vi "fitting.vi"() -> ()   [LabVIEW 2021]
uses:
  <vilib>/Utility/file.llb/Read Delimited Spreadsheet (DBL).vi
  <vilib>/Analysis/NI_AALPro.lvlib
panel:
  out "XY Graph 2":T1(graph)
  in  "path 2":path
  out "XY Graph":T1(graph)
  in  "path":path
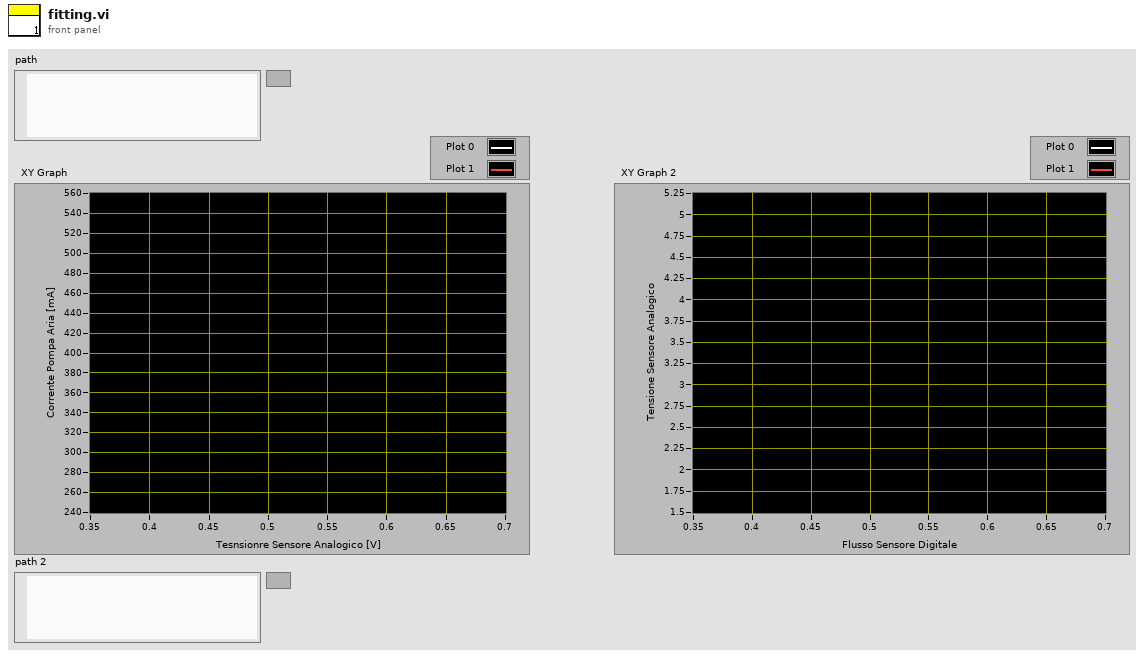
[diagram p1: front panel]
types:
  T1 = cluster{"all rows":dbl[], "Best Polynomial Fit":dbl[]}[]
  T2 = cluster{"all rows":dbl[], "Best Linear Fit":dbl[]}
  T3 = cluster{"all rows":dbl[], "Best Polynomial Fit":dbl[]}
  T4 = cluster{"all rows":dbl[], "Best Linear Fit":dbl[]}[]
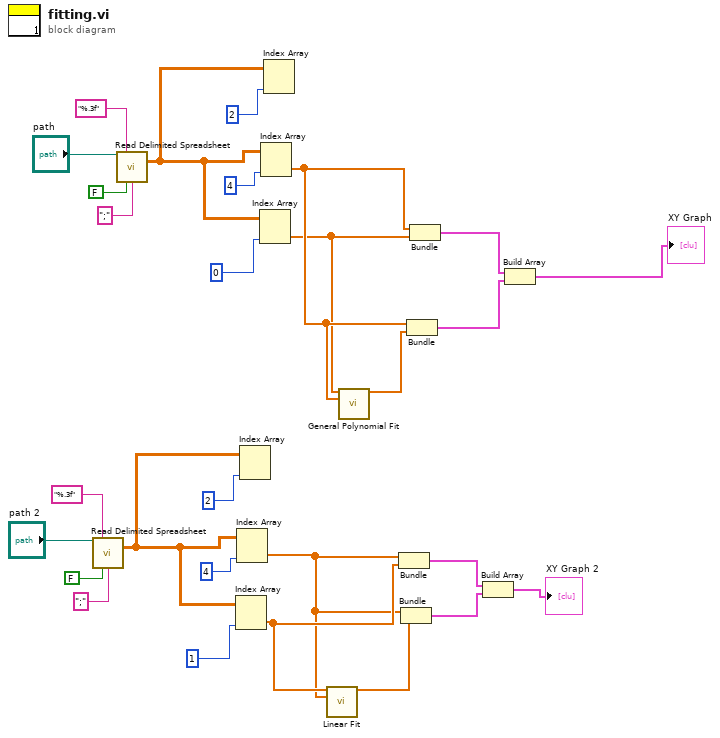
[diagram p0: block diagram]
diagram:
  n1 = call-poly <vilib>:"Read Delimited Spreadsheet.vi"("file path (dialog if empty)"="path 2", "format (%.3f)"="%.3f", "transpose? (F)"=FALSE, "delimiter (\\t)"=";" ("delimiter (\\t)")) -> ("all rows"=w14:dbl[][])  [unwired: 6 in, 5 out]
  n2 = call-poly <vilib>:"Read Delimited Spreadsheet.vi"("file path (dialog if empty)"="path", "format (%.3f)"="%.3f", "transpose? (F)"=FALSE, "delimiter (\\t)"=";" ("delimiter (\\t)")) -> ("all rows"=w21:dbl[][])  [unwired: 6 in, 5 out]
  n3 = Index Array(array=w14, index (col)=1 ("index")) -> (element=w6:dbl[])  [unwired: 1 in]
  n4 = Index Array(array=w14, index (col)=4 ("index")) -> (element=w5:dbl[])  [unwired: 1 in]
  n5 = Index Array(array=w14, index (col)=2 ("index")) -> ()  [unwired: 1 in, 1 out]
  n6 = Index Array(array=w21, index (col)=0 ("index")) -> (element=w17:dbl[])  [unwired: 1 in]
  n7 = Index Array(array=w21, index (col)=4 ("index")) -> (element=w18:dbl[])  [unwired: 1 in]
  n8 = Index Array(array=w21, index (col)=2 ("index")) -> ()  [unwired: 1 in, 1 out]
  n9 = call <vilib>:"Linear Fit.vi"("Y"=w6, "X"=w5) -> ("Best Linear Fit"=w4:dbl[])  [unwired: 9 in, 4 out]
  n10 = call <vilib>:"General Polynomial Fit.vi"("Y"=w17, "X"=w18) -> ("Best Polynomial Fit"=w16:dbl[])  [unwired: 10 in, 3 out]
  n11 = Bundle("all rows"=w5, "all rows"=w6) -> (w3:cluster{"all rows":dbl[], "all rows":dbl[]})  [unwired: 1 in]
  n12 = Bundle("all rows"=w5, "Best Linear Fit"=w4) -> (w2:T2)  [unwired: 1 in]
  n13 = Bundle("all rows"=w18, "Best Polynomial Fit"=w16) -> (w19:T3)  [unwired: 1 in]
  n14 = Bundle("all rows"=w18, "all rows"=w17) -> (w20:cluster{"all rows":dbl[], "all rows":dbl[]})  [unwired: 1 in]
  n15 = Build Array(w3, w2) -> (→"XY Graph 2":T4)
  n16 = Build Array(w20, w19) -> (→"XY Graph":T1)
